vi "读取注册表值.vi"(8 "value":string caption="子项", 9 "subkeyName":string caption="主项") -> (3 "Data":string caption="值")   [LabVIEW 2018]
doc: "本VI可能仅适用于Windows。\n\n本范例演示了从Wndows注册表读取数据的方式。运行本VI前必须先运行Write To Windows Registry.vi"
uses:
  <vilib>/registry/registry.llb/Registry RtKey.ctl
  <vilib>/registry/registry.llb/Read Registry Value Simple STR.vi
panel:
  out "error out":errorcluster caption="错误输出"
  # "本VI可能仅适用于Windows。\n\n本范例演示了从Wndows注册表读取数据的方式。运行本VI前必须先运行Write To Windows Registry.vi。"
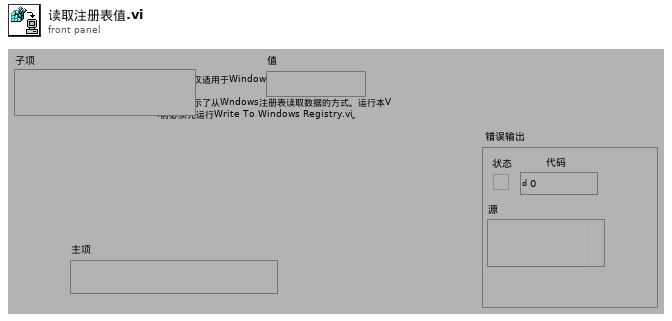
[diagram p1: front panel]
types:
  T1 = typedef "Registry RtKey.ctl" = enum32{"HKEY_CLASSES_ROOT", "HKEY_CURRENT_USER", "HKEY_LOCAL_MACHINE", "HKEY_USERS", "HKEY_PERFORMANCE_DATA", "HKEY_CURRENT_CONFIG", "HKEY_DYN_DATA"}
  T2 = typedef "Registry refnum.ctl" = refnum<k1>
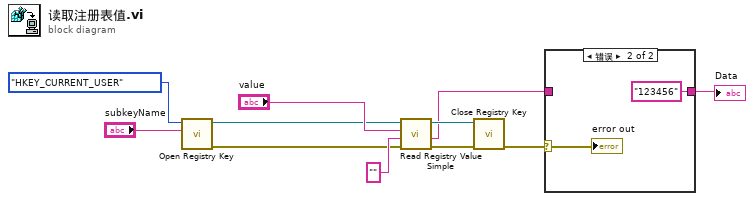
[diagram p0: block diagram]
diagram:
  n1 = call <vilib>:"Open Registry Key.vi"("subkey"="subkeyName", "root key (HKEY_LOCAL_MACHINE)"=Registry_RtKey."HKEY_CURRENT_USER") -> ("error out"=w4:errorcluster, "refnum out"=w5:T2)  [unwired: 8 in]
  n2 = call-poly <vilib>:"Read Registry Value Simple.vi"("error in (no error)"=w4, "default data"="", "value"="value", "refnum"=w5) -> ("error out"=w8:errorcluster, "String/Binary data"=w2:string, "refnum out"=w10:T2)  [unwired: 2 in, 1 out]
  n3 = call <vilib>:"Close Registry Key.vi"("error in (no error)"=w8, "refnum"=w10) -> ("error out"=w3:errorcluster)  [unwired: 5 in]
  n4 = case shown="错误" w3 {
    selector: w3 -> [_ w13]
    tunnel: w2 -> [w12 _]
    tunnel: [w12 "123456" ("String/Binary data")] -> w1
    frame No Error {
    }
    frame Error {
      "error out" <- w13
    }
  }
  "Data" <- w1
